vi "Validate.vi"(8 "error in (no error)":errorcluster, 10 "Loaded Settings":refnum<class "Settings Service.lvclass">, 11 "Settings Service in":refnum<class "Settings Service.lvclass">) -> (0 "error out":errorcluster, 3 "Settings Service out":refnum<class "Settings Service.lvclass">)   [LabVIEW 2026, in "Settings Service.lvclass"]
uses:
  Settings Service.lvclass
  Settings Service.lvclass/Settings Service.ctl
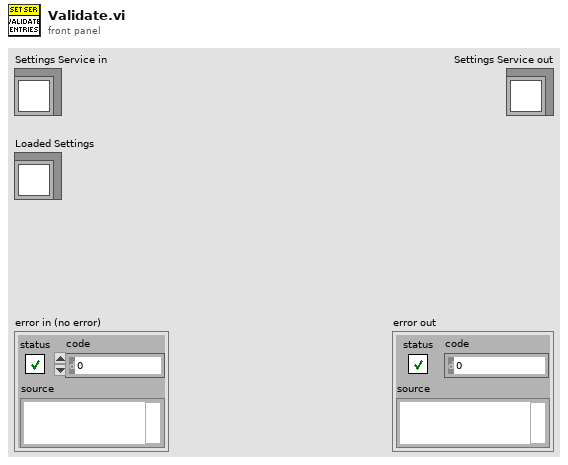
[diagram p1: front panel]
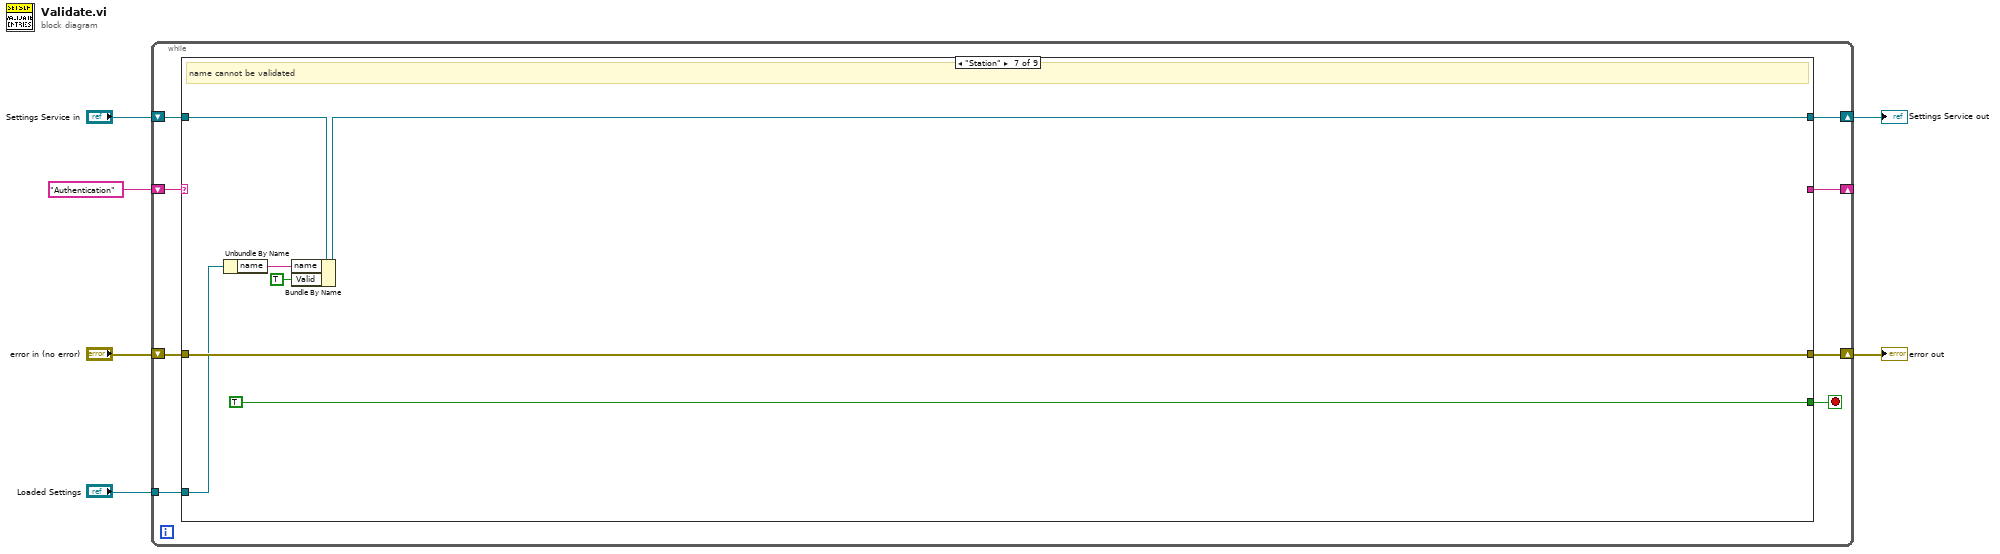
[diagram p0: block diagram]
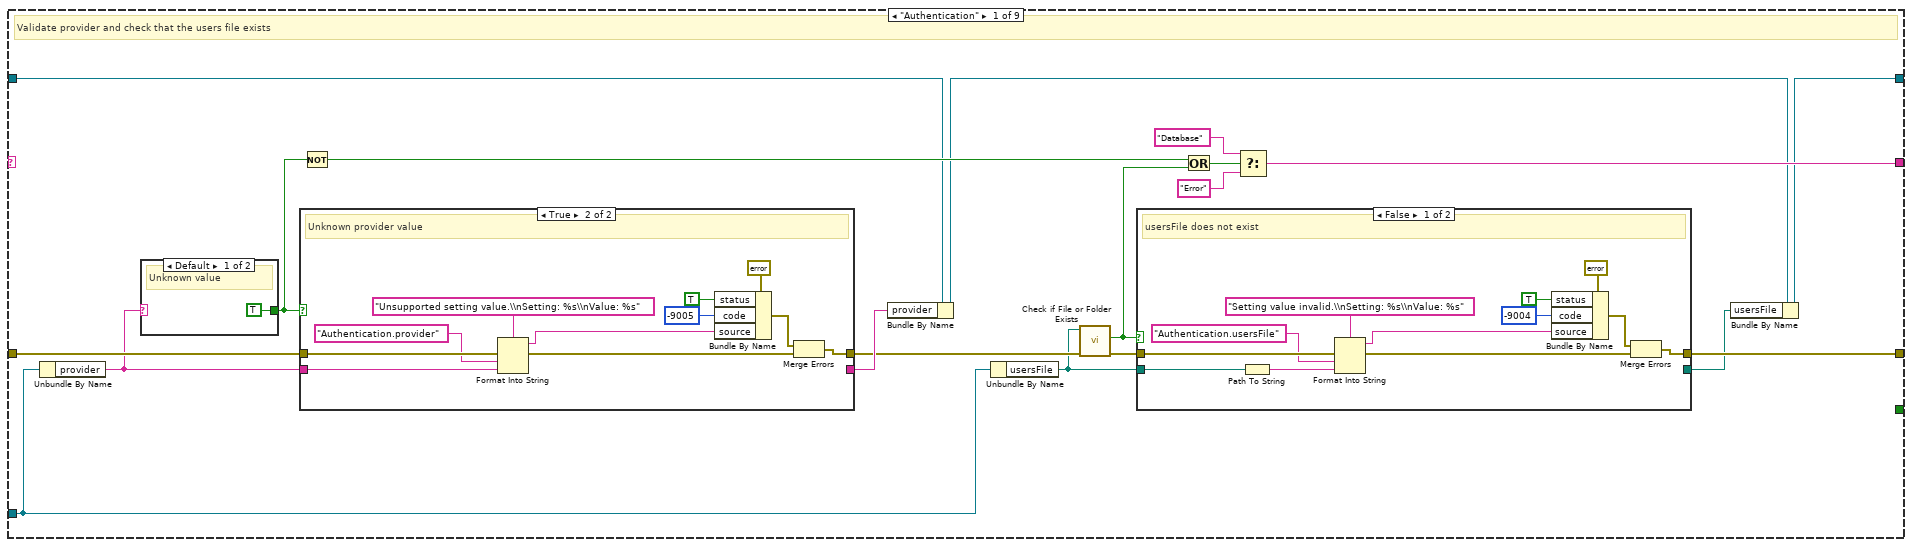
[diagram p2: hidden frame]
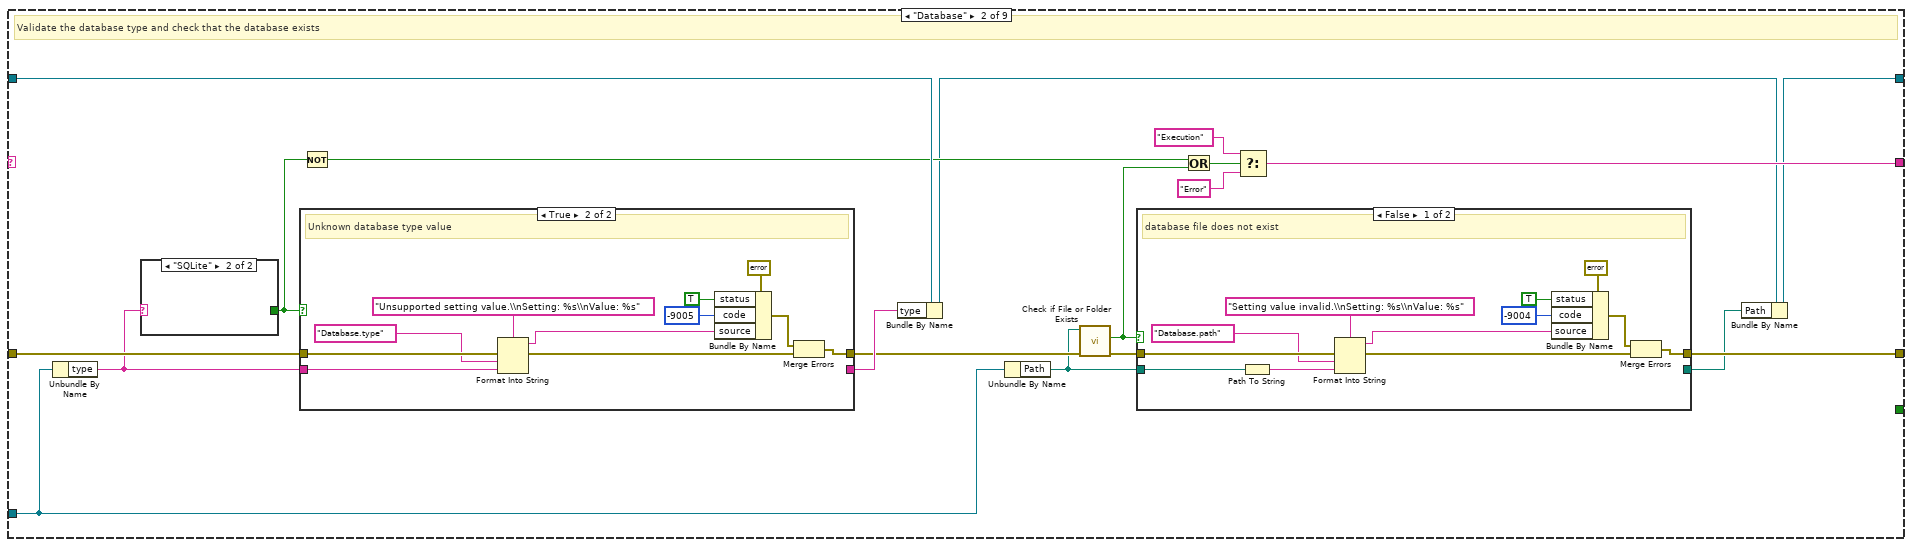
[diagram p6: hidden frame]
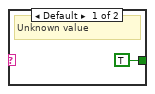
[diagram p9: hidden frame]
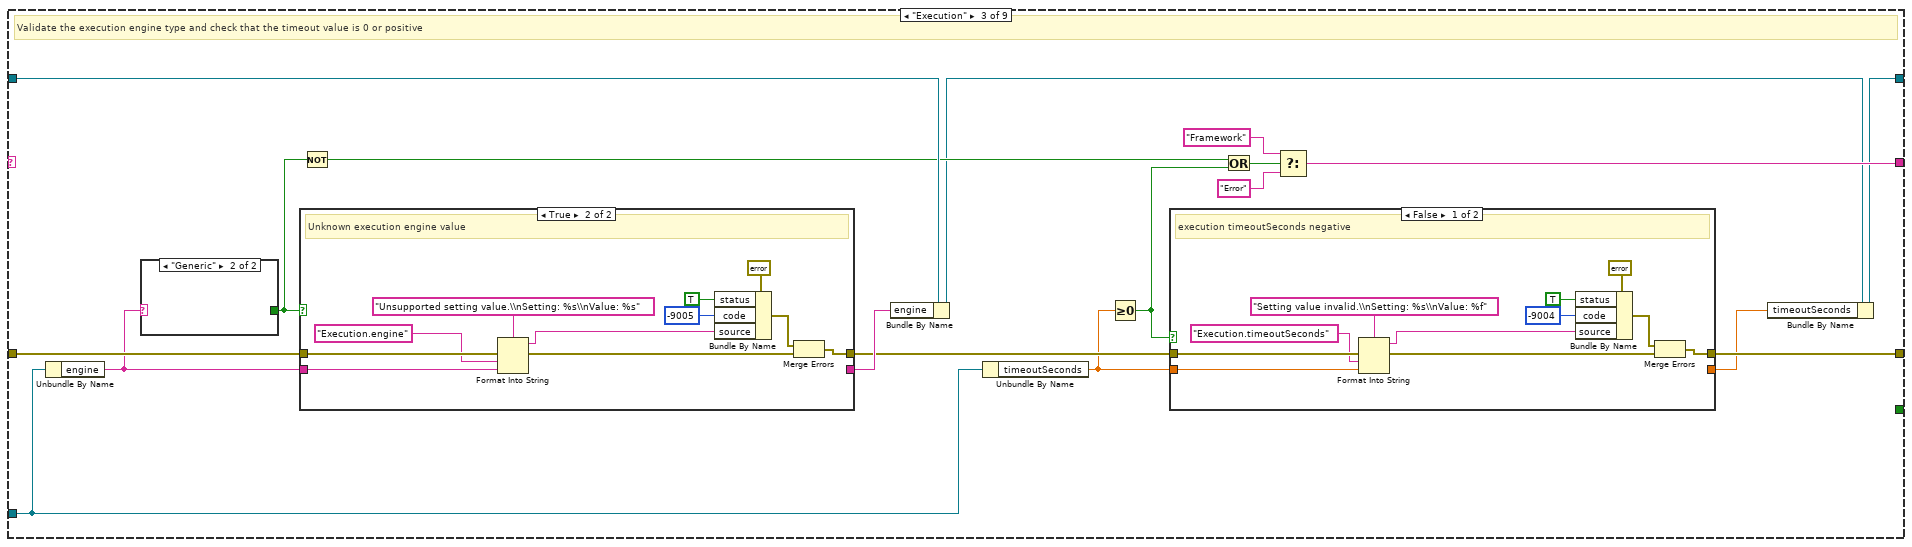
[diagram p10: hidden frame]
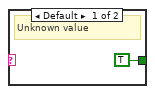
[diagram p13: hidden frame]
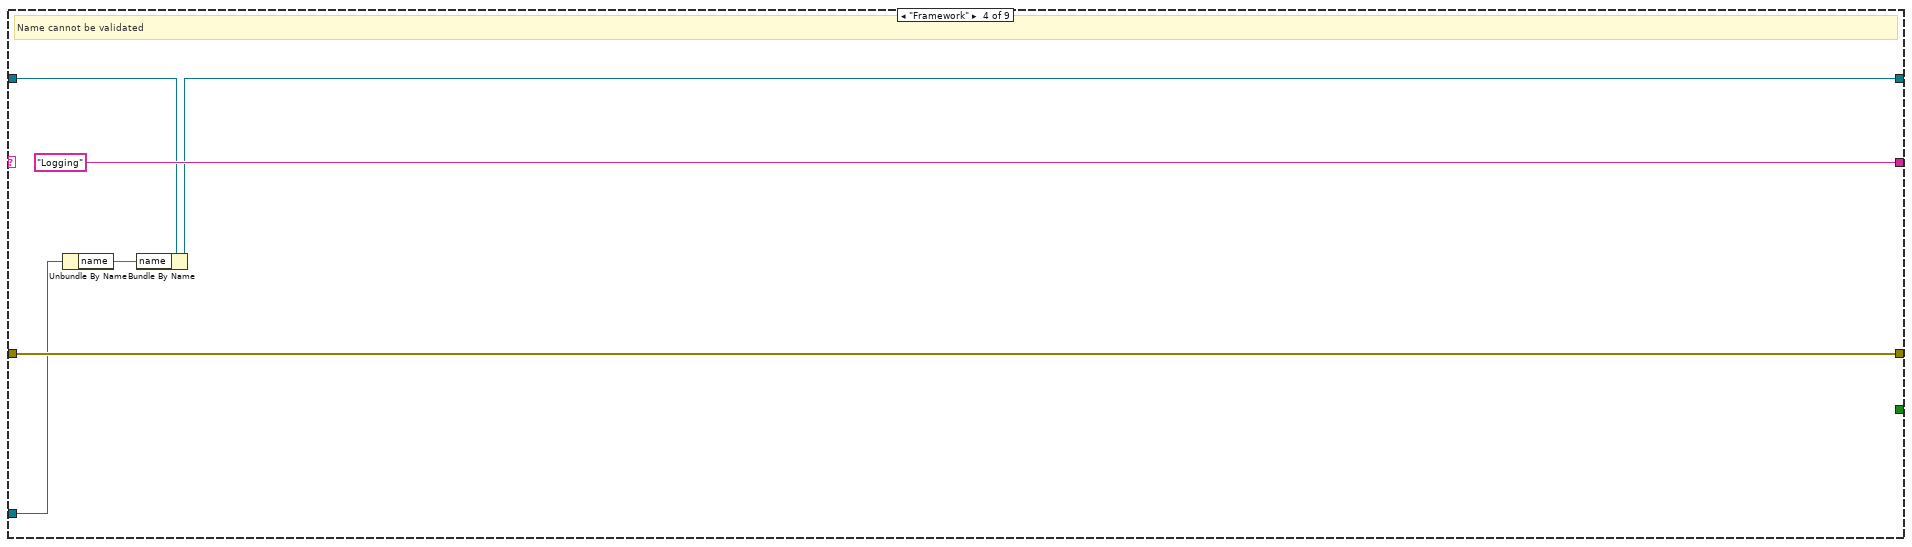
[diagram p14: hidden frame]
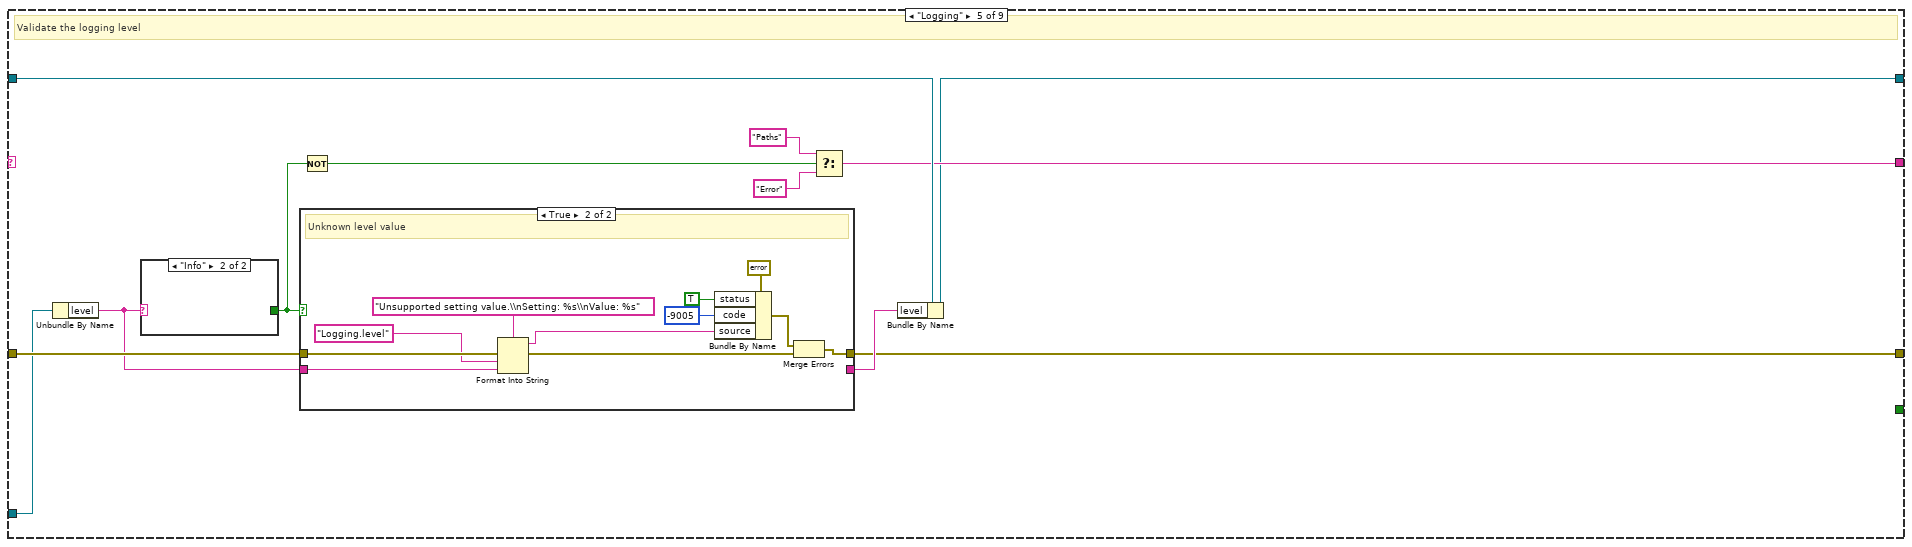
[diagram p15: hidden frame]
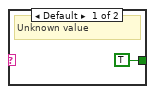
[diagram p17: hidden frame]
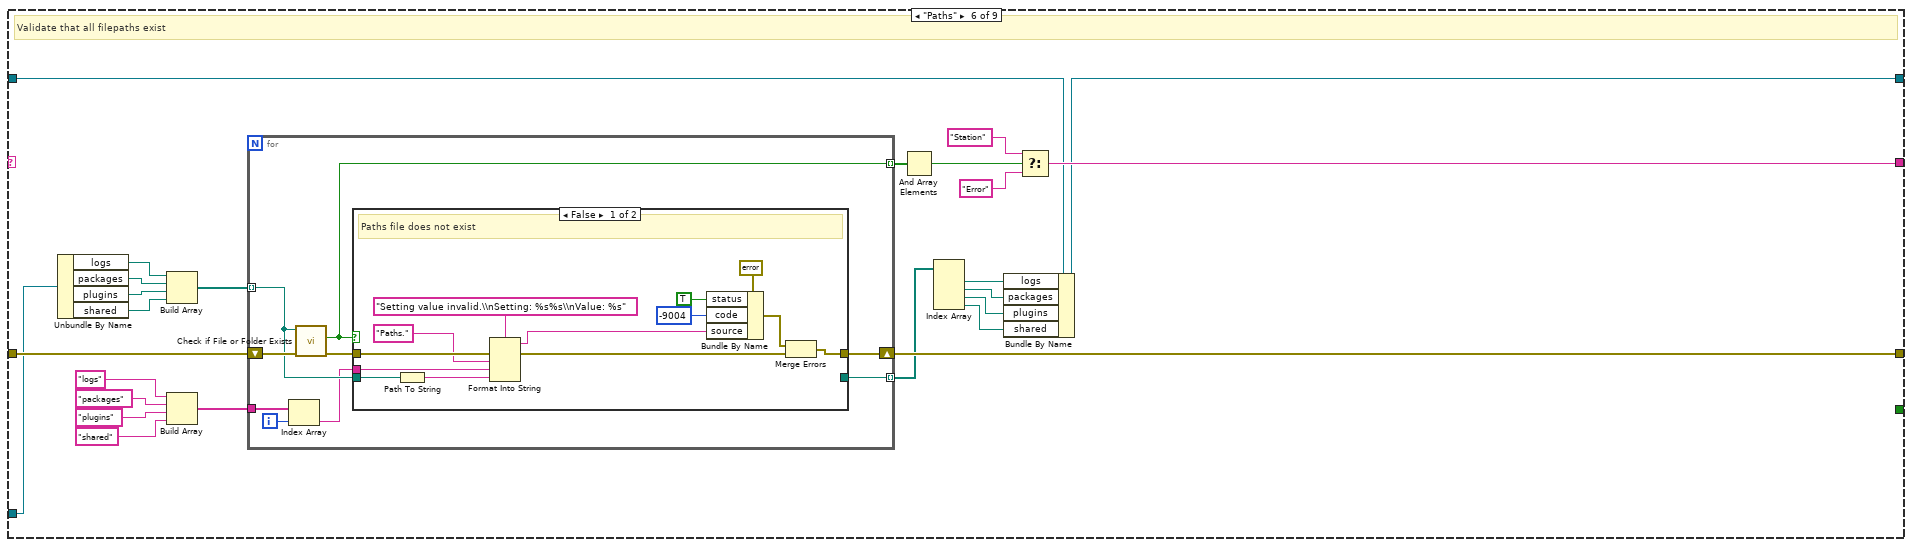
[diagram p18: hidden frame]
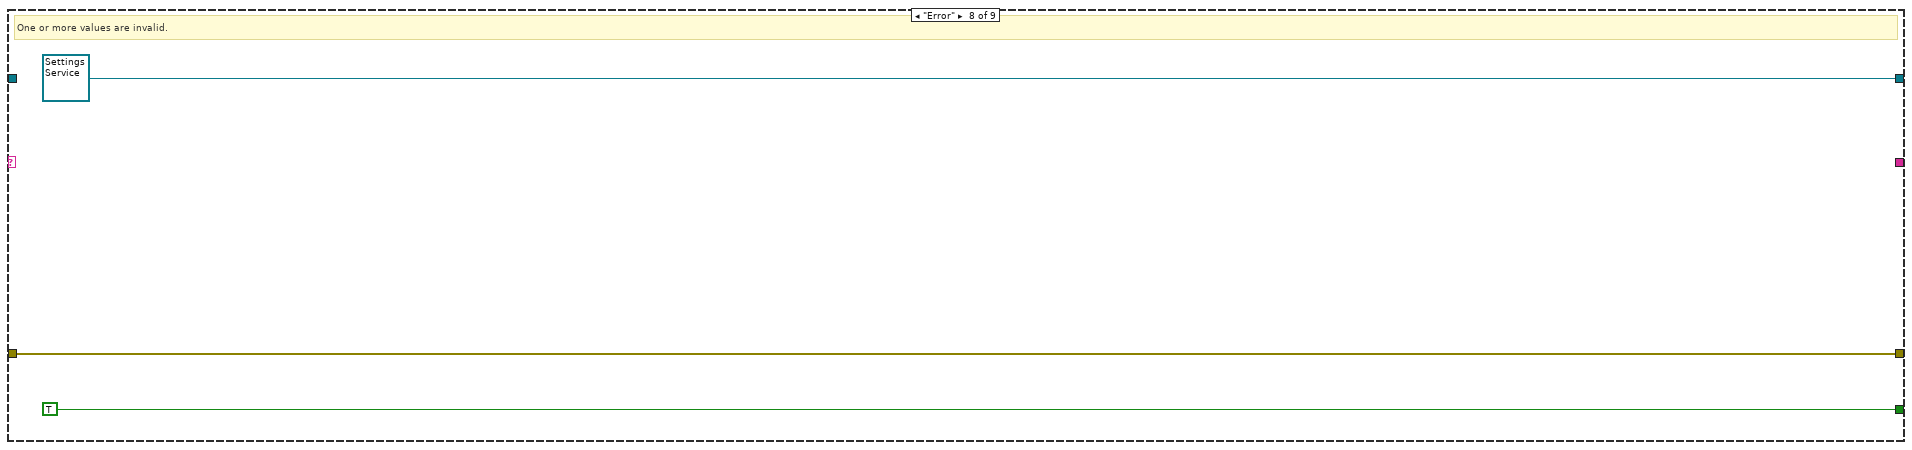
[diagram p20: hidden frame]
diagram:
  n1 = while {
    shift-right: [w10] -> _
    shift-left: "Authentication" -> [w14]
    shift-right: [w11] -> w3
    shift-left: "error in (no error)" -> [w12]
    shift-right: [w9] -> w2
    shift-left: "Settings Service in" -> [w13]
    tunnel: "Loaded Settings" -> [w7]
    stop <- w8 stop-if-true
    n2 = case shown="\"Station\"" w14 {
      tunnel: w13 -> [w16 w76 w123 w157 w168 w204 w239 _ w245]
      tunnel: w12 -> [w33 w80 w126 w159 w171 w203 w241 w244 w247]
      tunnel: [w21 w67 w116 w159 w161 w206 w241 w244 w247] -> w11
      tunnel: [w22 w68 w117 "Logging" ("f") w163 w207 _ _ _] -> w10
      tunnel: [w17 w63 w113 w155 w162 w205 w238 refnum<class "Settings Service.lvclass"> refnum ("Settings Service in") w245] -> w9
      tunnel: [_ _ _ _ _ _ TRUE TRUE TRUE] -> w8
      tunnel: w7 -> [w15 w62 w109 w156 w160 w186 w237 _ _]
      frame "Authentication" {
        # "Validate provider and check that the users file exists"
        n3 = Unbundle By Name(w15) -> ("provider"=w32:string)
        n4 = case shown="Default" w32 {
          tunnel: [TRUE _] -> w27
          frame Default {
            # "Unknown value"
          }
          frame "LocalFile" {
          }
        }
        n5 = case shown="True" w27 {
          tunnel: w33 -> [w49 w56]
          tunnel: w32 -> [w48 w51]
          tunnel: [w49 w50] -> w30
          tunnel: [w48 _] -> w31
          frame False {
            # "Valid provider value"
          }
          frame True {
            # "Unknown provider value"
            n6 = Format Into String(format string="Unsupported setting value.\\nSetting: %s\\nValue: %s", error in=w56, "Authentication.provider", w51) -> (resulting string=w53:string, error out=w55:errorcluster)  [unwired: 1 in]
            n7 = Bundle By Name(cluster=errorcluster {"status"=FALSE, "code"=0, "source"=""} ("error out"), "status"=TRUE, "code"=-9005, "source"=w53) -> (w57:errorcluster)
            n8 = Merge Errors(w57, w55) -> (w50:errorcluster)
          }
        }
        n9 = Not(x=w27) -> (.not. x?=w26:bool)
        n10 = Bundle By Name(cluster=w16, "provider"=w31) -> (w20:refnum<class "Settings Service.lvclass">)
        n11 = Unbundle By Name(w15) -> ("usersFile"=w19:path)
        n12 = call <vilib>:"Check if File or Folder Exists.vi"("error in (no error)"=w30, "path"=w19) -> ("error out"=w29:errorcluster, "file or folder exists?"=w28:bool)  [unwired: 7 in, 1 out]
        n13 = case shown="False" w28 {
          tunnel: w29 -> [w41 w47]
          tunnel: [w36 w47] -> w21
          tunnel: w19 -> [w35 w46]
          tunnel: [_ w46] -> w18
          frame False {
            # "usersFile does not exist"
            n14 = Path To String(path=w35) -> (string=w34:string)
            n15 = Format Into String(format string="Setting value invalid.\\nSetting: %s\\nValue: %s", error in=w41, "Authentication.usersFile", w34) -> (resulting string=w38:string, error out=w40:errorcluster)  [unwired: 1 in]
            n16 = Bundle By Name(cluster=errorcluster {"status"=FALSE, "code"=0, "source"=""} ("error out"), "status"=TRUE, "code"=-9004, "source"=w38) -> (w42:errorcluster)
            n17 = Merge Errors(w42, w40) -> (w36:errorcluster)
          }
          frame True {
            # "Valid usersFile value"
          }
        }
        n18 = Or(x=w26, y=w28) -> (x .or. y?=w25:bool)
        n19 = Select(t="Database", s=w25, f="Error") -> (s? t:f=w22:string)
        n20 = Bundle By Name(cluster=w20, "usersFile"=w18) -> (w17:refnum<class "Settings Service.lvclass">)
      }
      frame "Database" {
        # "Validate the database type and check that the database exists"
        n21 = Unbundle By Name(w62) -> ("type"=w79:string)
        n22 = case shown="\"SQLite\"" w79 {
          tunnel: [TRUE _] -> w73
          frame Default {
            # "Unknown value"
          }
          frame "SQLite" {
          }
        }
        n23 = case shown="True" w73 {
          tunnel: w80 -> [w96 w103]
          tunnel: w79 -> [w95 w98]
          tunnel: [w96 w97] -> w77
          tunnel: [w95 _] -> w78
          frame False {
            # "Valid database type value"
          }
          frame True {
            # "Unknown database type value"
            n24 = Format Into String(format string="Unsupported setting value.\\nSetting: %s\\nValue: %s", error in=w103, "Database.type", w98) -> (resulting string=w100:string, error out=w102:errorcluster)  [unwired: 1 in]
            n25 = Bundle By Name(cluster=errorcluster {"status"=FALSE, "code"=0, "source"=""} ("error out"), "status"=TRUE, "code"=-9005, "source"=w100) -> (w104:errorcluster)
            n26 = Merge Errors(w104, w102) -> (w97:errorcluster)
          }
        }
        n27 = Not(x=w73) -> (.not. x?=w72:bool)
        n28 = Bundle By Name(cluster=w76, "type"=w78) -> (w66:refnum<class "Settings Service.lvclass">)
        n29 = Unbundle By Name(w62) -> ("Path"=w65:path)
        n30 = call <vilib>:"Check if File or Folder Exists.vi"("error in (no error)"=w77, "path"=w65) -> ("error out"=w75:errorcluster, "file or folder exists?"=w74:bool)  [unwired: 7 in, 1 out]
        n31 = case shown="False" w74 {
          tunnel: w75 -> [w88 w94]
          tunnel: [w83 w94] -> w67
          tunnel: w65 -> [w82 w93]
          tunnel: [_ w93] -> w64
          frame False {
            # "database file does not exist"
            n32 = Path To String(path=w82) -> (string=w81:string)
            n33 = Format Into String(format string="Setting value invalid.\\nSetting: %s\\nValue: %s", error in=w88, "Database.path", w81) -> (resulting string=w85:string, error out=w87:errorcluster)  [unwired: 1 in]
            n34 = Bundle By Name(cluster=errorcluster {"status"=FALSE, "code"=0, "source"=""} ("error out"), "status"=TRUE, "code"=-9004, "source"=w85) -> (w89:errorcluster)
            n35 = Merge Errors(w89, w87) -> (w83:errorcluster)
          }
          frame True {
            # "Valid database path value"
          }
        }
        n36 = Or(x=w72, y=w74) -> (x .or. y?=w71:bool)
        n37 = Select(t="Execution", s=w71, f="Error") -> (s? t:f=w68:string)
        n38 = Bundle By Name(cluster=w66, "Path"=w64) -> (w63:refnum<class "Settings Service.lvclass">)
      }
      frame "Execution" {
        # "Validate the execution engine type and check that the timeout value is 0 or positive"
        n39 = Unbundle By Name(w109) -> ("engine"=w125:string)
        n40 = case shown="\"Generic\"" w125 {
          tunnel: [TRUE _] -> w122
          frame Default {
            # "Unknown value"
          }
          frame "Generic" {
          }
        }
        n41 = case shown="True" w122 {
          tunnel: w126 -> [w141 w148]
          tunnel: w125 -> [w140 w143]
          tunnel: [w141 w142] -> w112
          tunnel: [w140 _] -> w124
          frame False {
            # "Valid execution engine value"
          }
          frame True {
            # "Unknown execution engine value"
            n42 = Format Into String(format string="Unsupported setting value.\\nSetting: %s\\nValue: %s", error in=w148, "Execution.engine", w143) -> (resulting string=w145:string, error out=w147:errorcluster)  [unwired: 1 in]
            n43 = Bundle By Name(cluster=errorcluster {"status"=FALSE, "code"=0, "source"=""} ("error out"), "status"=TRUE, "code"=-9005, "source"=w145) -> (w149:errorcluster)
            n44 = Merge Errors(w149, w147) -> (w142:errorcluster)
          }
        }
        n45 = Not(x=w122) -> (.not. x?=w121:bool)
        n46 = Bundle By Name(cluster=w123, "engine"=w124) -> (w115:refnum<class "Settings Service.lvclass">)
        n47 = Unbundle By Name(w109) -> ("timeoutSeconds"=w111:dbl)
        n48 = Greater Or Equal To 0?(x=w111) -> (x >= 0?=w110:bool)
        n49 = case shown="False" w110 {
          tunnel: w112 -> [w133 w139]
          tunnel: [w128 w139] -> w116
          tunnel: w111 -> [w127 w138]
          tunnel: [_ w138] -> w114
          frame False {
            # "execution timeoutSeconds negative"
            n50 = Format Into String(format string="Setting value invalid.\\nSetting: %s\\nValue: %f", error in=w133, "Execution.timeoutSeconds", w127) -> (resulting string=w130:string, error out=w132:errorcluster)  [unwired: 1 in]
            n51 = Bundle By Name(cluster=errorcluster {"status"=FALSE, "code"=0, "source"=""} ("error out"), "status"=TRUE, "code"=-9004, "source"=w130) -> (w134:errorcluster)
            n52 = Merge Errors(w134, w132) -> (w128:errorcluster)
          }
          frame True {
            # "Valid execution timeoutSeconds value"
          }
        }
        n53 = Or(x=w121, y=w110) -> (x .or. y?=w120:bool)
        n54 = Select(t="Framework", s=w120, f="Error") -> (s? t:f=w117:string)
        n55 = Bundle By Name(cluster=w115, "timeoutSeconds"=w114) -> (w113:refnum<class "Settings Service.lvclass">)
      }
      frame "Framework" {
        # "Name cannot be validated"
        n56 = Unbundle By Name(w156) -> ("name"=w154:string)
        n57 = Bundle By Name(cluster=w157, "name"=w154) -> (w155:refnum<class "Settings Service.lvclass">)
      }
      frame "Logging" {
        # "Validate the logging level"
        n58 = Unbundle By Name(w160) -> ("level"=w170:string)
        n59 = case shown="\"Info\"" w170 {
          tunnel: [TRUE _] -> w167
          frame Default {
            # "Unknown value"
          }
          frame "Info" {
          }
        }
        n60 = case shown="True" w167 {
          tunnel: w171 -> [w173 w180]
          tunnel: w170 -> [w172 w175]
          tunnel: [w173 w174] -> w161
          tunnel: [w172 _] -> w169
          frame False {
            # "Valid level value"
          }
          frame True {
            # "Unknown level value"
            n61 = Format Into String(format string="Unsupported setting value.\\nSetting: %s\\nValue: %s", error in=w180, "Logging.level", w175) -> (resulting string=w177:string, error out=w179:errorcluster)  [unwired: 1 in]
            n62 = Bundle By Name(cluster=errorcluster {"status"=FALSE, "code"=0, "source"=""} ("error out"), "status"=TRUE, "code"=-9005, "source"=w177) -> (w181:errorcluster)
            n63 = Merge Errors(w181, w179) -> (w174:errorcluster)
          }
        }
        n64 = Not(x=w167) -> (.not. x?=w166:bool)
        n65 = Select(t="Paths", s=w166, f="Error") -> (s? t:f=w163:string)
        n66 = Bundle By Name(cluster=w168, "level"=w169) -> (w162:refnum<class "Settings Service.lvclass">)
      }
      frame "Paths" {
        # "Validate that all filepaths exist"
        n67 = Unbundle By Name(w186) -> ("logs"=w202:path, "packages"=w201:path, "plugins"=w200:path, "shared"=w199:path)
        n68 = Build Array(w202, w201, w200, w199) -> (w198:path[])
        n69 = Build Array("logs", "packages", "plugins", "shared") -> (w193:string[])
        n70 = for {
          tunnel: [w218] -> w210 mode=indexing
          tunnel: [w216] -> w192 mode=indexing
          shift-right: [w217] -> w206
          shift-left: w203 -> [w215]
          tunnel: w198 -> [w214] mode=indexing
          tunnel: w193 -> [w213]
          i -> [w212]
          n71 = Index Array(array=w213, index=w212) -> (element=w211:string)
          n72 = call <vilib>:"Check if File or Folder Exists.vi"("error in (no error)"=w215, "path"=w214) -> ("error out"=w219:errorcluster, "file or folder exists?"=w218:bool)  [unwired: 7 in, 1 out]
          n73 = case shown="False" w218 {
            tunnel: w219 -> [w228 w234]
            tunnel: [w223 w234] -> w217
            tunnel: w214 -> [w222 w233]
            tunnel: [_ w233] -> w216
            tunnel: w211 -> [w220 _]
            frame False {
              # "Paths file does not exist"
              n74 = Path To String(path=w222) -> (string=w221:string)
              n75 = Format Into String(format string="Setting value invalid.\\nSetting: %s%s\\nValue: %s", error in=w228, "Paths.", w220, w221) -> (resulting string=w225:string, error out=w227:errorcluster)  [unwired: 1 in]
              n76 = Bundle By Name(cluster=errorcluster {"status"=FALSE, "code"=0, "source"=""} ("error out"), "status"=TRUE, "code"=-9004, "source"=w225) -> (w229:errorcluster)
              n77 = Merge Errors(w229, w227) -> (w223:errorcluster)
            }
            frame True {
              # "Valid path value"
            }
          }
        }
        n78 = And Array Elements(Boolean array=w210) -> (logical AND=w191:bool)
        n79 = Index Array(array=w192) -> (element #1=w190:path, element #2=w189:path, element #3=w188:path, element #4=w187:path)  [unwired: 4 in]
        n80 = Bundle By Name(cluster=w204, "logs"=w190, "packages"=w189, "plugins"=w188, "shared"=w187) -> (w205:refnum<class "Settings Service.lvclass">)
        n81 = Select(t="Station", s=w191, f="Error") -> (s? t:f=w207:string)
      }
      frame "Station" {
        # "name cannot be validated"
        n82 = Unbundle By Name(w237) -> ("name"=w236:string)
        n83 = Bundle By Name(cluster=w239, "name"=w236, "Valid"=TRUE) -> (w238:refnum<class "Settings Service.lvclass">)
      }
      frame "Error" {
        # "One or more values are invalid."
      }
      frame Default {
        # "Unknown case"
      }
    }
  }
  "Settings Service out" <- w2
  "error out" <- w3
